vi "Cuboids example.vi"() -> ()   [LabVIEW 2013]
uses:
  Cuboids sub vis/Cuboid properties.ctl
  <vilib>/Utility/miscctls.llb/LV3DPointTypeDef.ctl
  <vilib>/Analysis/baseanly.llb/A x Vector.vi
  <vilib>/Analysis/_algsub.llb/Vector Norm.vi
  <vilib>/Analysis/_algsub.llb/Real Vector Norm.vi
  <vilib>/Analysis/baseanly.llb/Unit Vector.vi
  <vilib>/Analysis/baseanly.llb/Unit Vector (DBL).vi
  <vilib>/Analysis/baseanly.llb/Dot Product.vi
  <vilib>/Analysis/baseanly.llb/Real Dot Product.vi
  Cuboids sub vis/2D cross product.vi
  <vilib>/picture/3D Picture Control/Object/Add Object (no reference).vi
  <vilib>/picture/3D Picture Control/Object/Create Object (name).vi
  <vilib>/Analysis/Matrix/Numeric/Conversions/Array To Matrix - RA2.vi
  <vilib>/picture/3D Picture Control/NI_3D Picture Control.lvlib
  <vilib>/Analysis/NI_AALBase.lvlib
  <vilib>/Analysis/Matrix/NI_Matrix.lvlib
panel:
  in  "Reset view":bool
  in  "Stop Button":bool
  out "error out":errorcluster
  in  "Circle test min. dist.":dbl=100.0
  out "Minimum separation":dbl=0.19883626783883718
  out "Collision":bool
  in  "Rz2 (deg)":sgl(knob)=290.0 min=0 max=360 step=1 scale=0.0..360.0
  in  "Tx2, Ty2, Tz2":sgl[](array[slide])=[1.0, 0.0, 0.0] min=-5 max=5 step=0.1 scale=-5.0..5.0
  in  "Lx2, Ly2, Lz2":sgl[](array[slide])=[2.0, 0.2, 0.2] min=0 max=5 step=0.1 scale=0.0..5.0
  in  "Lx1, Ly1, Lz1":sgl[](array[slide])=[1.0, 1.0, 1.0] min=0 max=5 scale=0.0..5.0
  out "World":refnum<vi>(3d-picture)
  # "PN 30/08/2014"
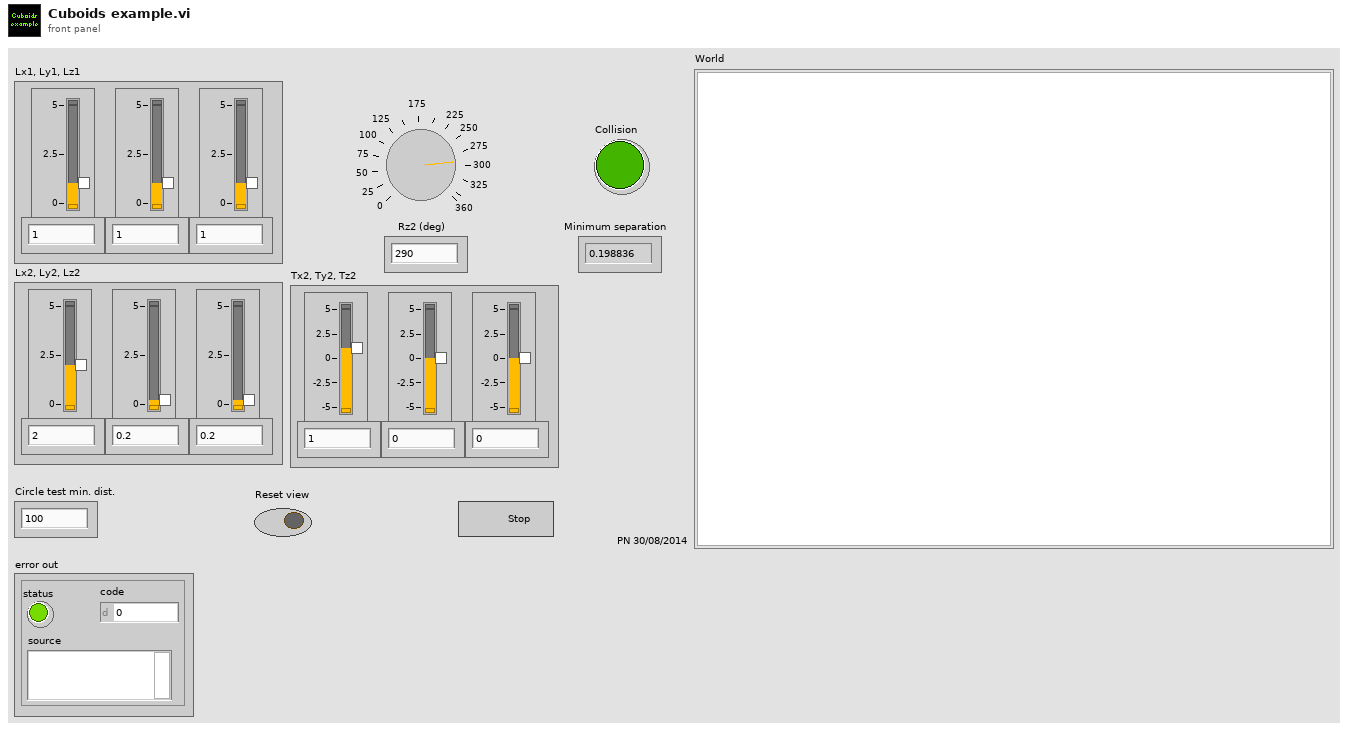
[diagram p1: front panel]
types:
  T1 = cluster{"Red":sgl, "Green":sgl, "Blue":sgl, "Alpha":sgl}
  T2 = typedef "LV3DPointTypeDef.ctl" = cluster{"X":sgl, "Y":sgl, "Z":sgl}
  T3 = typedef "Cuboid properties.ctl" = cluster{"Vertices (x, y)":dbl[][], "Zmin":dbl, "Zmax":dbl, "Centroid (x, y)":dbl[], "Radius":dbl, "Edge normals (x, y)":dbl[][], "Edge vectors (x, y)":dbl[][]}
  T4 = typedef "NI_Matrix.lvlib/RealMatrix.ctl" = dbl[][]
  T5 = cluster{"Vertical Pointer Slide":sgl, "Vertical Pointer Slide":sgl, "Vertical Pointer Slide":sgl}
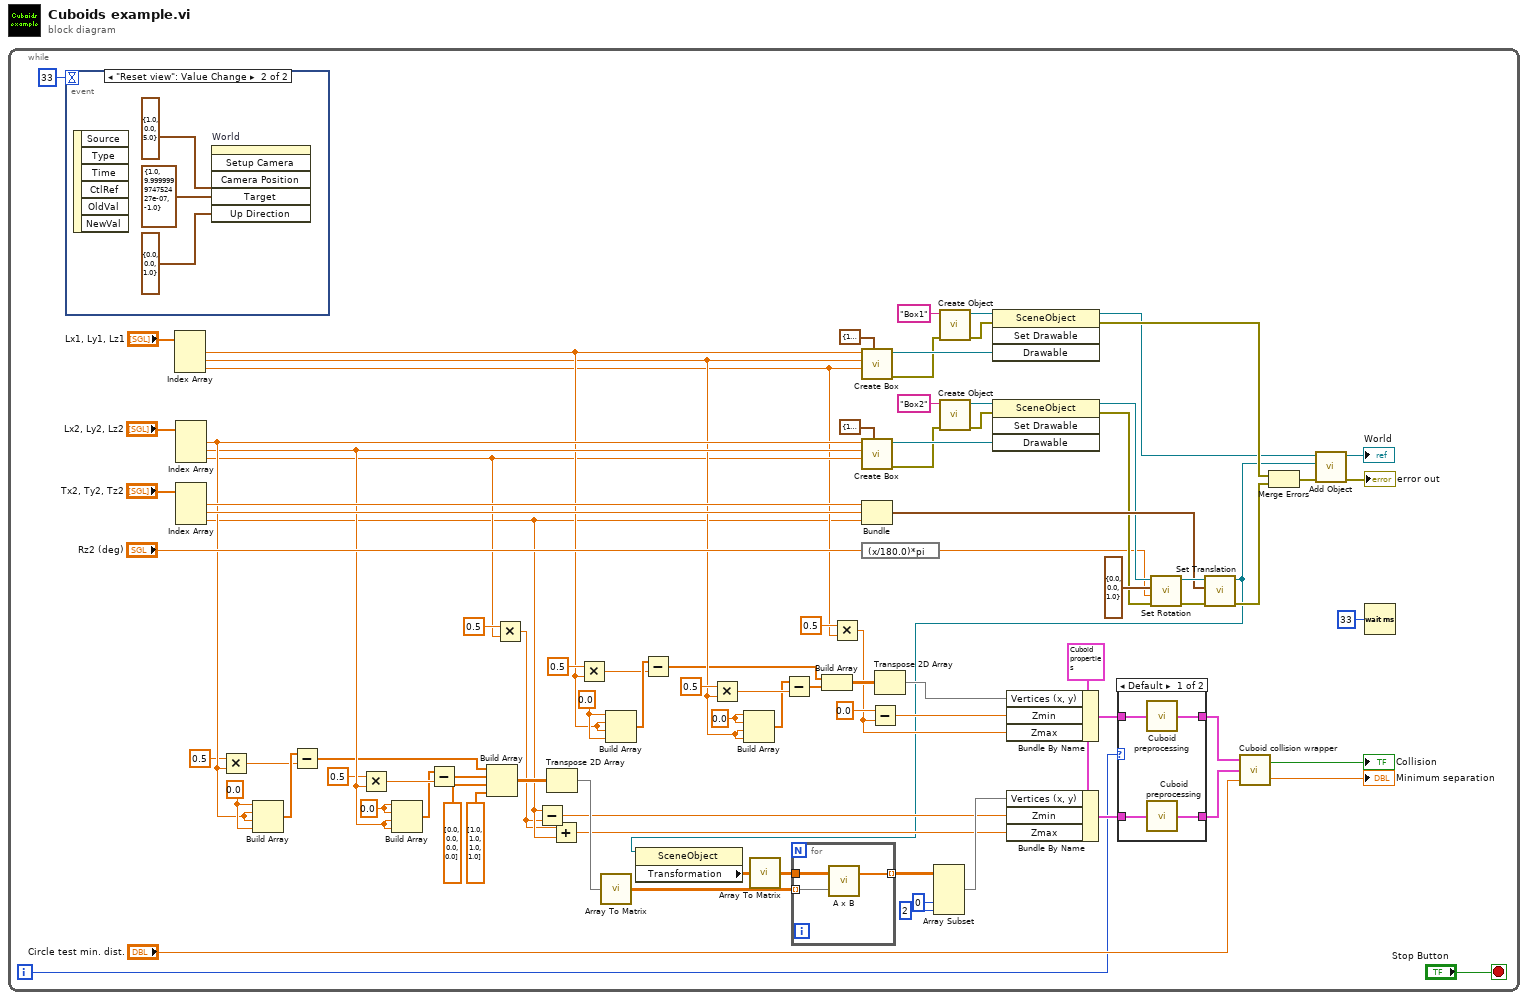
[diagram p0: block diagram]
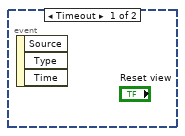
[diagram p2: hidden frame]
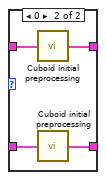
[diagram p3: hidden frame]
diagram:
  n1 = while {
    i -> [w16]
    stop <- "Stop Button" stop-if-true
    w53 = sgl 0.0 ("element")
    w54 = sgl 0.0 ("element")
    w55 = sgl 0.0 ("element")
    w56 = sgl 0.0 ("element")
    w67 = T3 {"Vertices (x, y)"=[[0.0, 0.0, 0.0], [1.0, 1.0, 0.0], [0.0, 1.0, 0.0], [1.0, 0.0, 0.0]], "Zmin"=0.0, "Zmax"=1.0, "Centroid (x, y)"=[0.0, 0.0, 0.0], "Radius"=0.0, "Edge normals (x, y)"=[[0.0, 0.0, 0.0], [0.0, 0.0, 0.0], [0.0, 0.0, 0.0], [0.0, 0.0, 0.0]], "Edge vectors (x, y)"=[[0.0, 0.0], [0.0, 0.0], [0.0, 0.0], [0.0, 0.0]]} ("Cuboid properties in")
    n2 = event shown="[1] \"Reset view\": Value Change" {
      selector: _ -> [_ _]
      dyn-events: _ -> [_ _]
      timeout: 33 -> [_ _]
      event Timeout {
        n3 = event-data() -> ()  [unwired: 1 in, 3 out]
      }
      event "Reset view": Value Change {
        n4 = event-data() -> ()  [unwired: 1 in, 6 out]
        n5 = invoke on="World" class="SceneGraphDisp (strict)" method="Setup Camera"("Camera Position"=T2 {"X"=1.0, "Y"=0.0, "Z"=5.0}, "Target"=T2 {"X"=1.0, "Y"=1e-06, "Z"=-1.0}, "Up Direction"=T2 {"X"=0.0, "Y"=0.0, "Z"=1.0}) -> ()  [unwired: 3 in, 6 out]
      }
    }
    n6 = Index Array(array="Lx1, Ly1, Lz1") -> (element #1=w33:sgl, element #2=w31:sgl, element #3=w9:sgl)  [unwired: 3 in]
    n7 = Index Array(array="Lx2, Ly2, Lz2") -> (element #1=w44:sgl, element #2=w42:sgl, element #3=w12:sgl)  [unwired: 3 in]
    n8 = Index Array(array="Tx2, Ty2, Tz2") -> (element #1=w64:sgl, element #2=w63:sgl, element #3=w5:sgl)  [unwired: 3 in]
    n9 = Multiply(x=sgl 0.5, y=w44) -> (x*y=w39:sgl)
    n10 = Build Array(w54, w44, w44, w54) -> (w40:sgl[])
    n11 = Subtract(x=w40, y=w39) -> (x-y=w38:sgl[])
    n12 = Multiply(x=sgl 0.5, y=w42) -> (x*y=w37:sgl)
    n13 = Build Array(w53, w53, w42, w42) -> (w36:sgl[])
    n14 = Subtract(x=w36, y=w37) -> (x-y=w35:sgl[])
    n15 = Build Array(w38, w35, sgl[] [0.0, 0.0, 0.0, 0.0], sgl[] [1.0, 1.0, 1.0, 1.0]) -> (w62:sgl[][])
    n16 = Multiply(x=sgl 0.5, y=w12) -> (x*y=w3:sgl)
    n17 = Subtract(x=w5, y=w3) -> (x-y=w4:sgl)
    n18 = Transpose 2D Array(2D array=w62) -> (transposed array=w24:sgl[][])
    n19 = Add(x=w3, y=w5) -> (x+y=w6:sgl)
    n20 = Multiply(x=sgl 0.5, y=w33) -> (x*y=w29:sgl)
    n21 = call-poly <vilib>:"Array To Matrix.vi"("Real 2D Array"=w24) -> ("Real Matrix"=w50:T4)
    n22 = Build Array(w56, w33, w33, w56) -> (w30:sgl[])
    n23 = Subtract(x=w30, y=w29) -> (x-y=w28:sgl[])
    n24 = Multiply(x=sgl 0.5, y=w31) -> (x*y=w27:sgl)
    n25 = Build Array(w55, w55, w31, w31) -> (w26:sgl[])
    n26 = Subtract(x=w26, y=w27) -> (x-y=w25:sgl[])
    n27 = Build Array(w28, w25) -> (w65:sgl[][])
    n28 = Multiply(x=sgl 0.5, y=w9) -> (x*y=w7:sgl)
    n29 = call <vilib>:"Create Box.vi"("Color"=T1 {"Red"=1.0, "Green"=1.0, "Blue"=1.0, "Alpha"=1.0}, "Length Z"=w9, "Length Y"=w31, "Length X"=w33) -> ("error out"=w82:errorcluster, "New Box Refnum"=w87:refnum<vi>)  [unwired: 6 in]
    n30 = call <vilib>:"Create Box.vi"("Color"=T1 {"Red"=1.0, "Green"=1.0, "Blue"=1.0, "Alpha"=1.0}, "Length Z"=w12, "Length Y"=w42, "Length X"=w44) -> ("error out"=w72:errorcluster, "New Box Refnum"=w83:refnum<vi>)  [unwired: 6 in]
    n31 = Bundle("Vertical Pointer Slide"=w64, "Vertical Pointer Slide"=w63, "Vertical Pointer Slide"=w5) -> (w79:T5)  [unwired: 1 in]
    n32 = expression code="(x/180.0)*pi" ("degrees to radians")("Rz2 (deg)") -> (w59:sgl)
    n33 = Subtract(x=sgl 0.0 ("element"), y=w7) -> (x-y=w8:sgl)
    n34 = Transpose 2D Array(2D array=w65) -> (transposed array=w61:sgl[][])
    n35 = call-poly <vilib>:"Create Object.vi"("error in (no error)"=w82, "Name"="Box1") -> ("error out"=w88:errorcluster, "Scene:New Object"=w89:refnum<vi>)  [unwired: 8 in]
    n36 = call-poly <vilib>:"Create Object.vi"("error in (no error)"=w72, "Name"="Box2") -> ("error out"=w71:errorcluster, "Scene:New Object"=w74:refnum<vi>)  [unwired: 8 in]
    n37 = invoke class="SceneObject" method="Set Drawable"(reference=w89, error in=w88, "Drawable"=w87) -> (reference out=w57:refnum<vi>, error out=w58:errorcluster)  [unwired: 1 in, 2 out]
    n38 = invoke class="SceneObject" method="Set Drawable"(reference=w74, error in=w71, "Drawable"=w83) -> (reference out=w75:refnum<vi>, error out=w76:errorcluster)  [unwired: 1 in, 2 out]
    n39 = Bundle By Name(cluster=w67, "Vertices (x, y)"=w61, "Zmin"=w8, "Zmax"=w7) -> (w68:T3)
    n40 = call <vilib>:"Set Rotation.vi"("error in (no error)"=w76, "Angle"=w59, "Axis"=cluster{"X":sgl, "Y":sgl, "Z":sgl} {"X"=0.0, "Y"=0.0, "Z"=1.0}, "Scene Object"=w75) -> ("error out"=w80:errorcluster, "Rotated Scene Object"=w81:refnum<vi>)  [unwired: 6 in]
    n41 = call <vilib>:"Set Translation.vi"("error in (no error)"=w80, "Translation"=w79, "Scene Object"=w81) -> ("error out"=w69:errorcluster, "Translated Object"=w1:refnum<vi>)  [unwired: 7 in]
    n42 = property class="SceneObject"(reference=w1) -> ("Transformation"=w52:sgl[][])  [unwired: 1 in, 2 out]
    n43 = call-poly <vilib>:"Array To Matrix.vi"("Real 2D Array"=w52) -> ("Real Matrix"=w17:T4)
    n44 = for {
      tunnel: w17 -> [w106]
      tunnel: w50 -> [w105] mode=indexing
      tunnel: [w104] -> w48 mode=indexing
      n45 = call-poly <vilib>:"A x B.vi"("Vector"=w105, "A"=w106) -> ("A x Vector"=w104:dbl[])  [unwired: 1 out]
    }
    n46 = Array Subset(array=w48, index (col)=0 ("index"), length (col)=2 ("length")) -> (w45:dbl[][])  [unwired: 2 in]
    n47 = Bundle By Name(cluster=w67, "Vertices (x, y)"=w45, "Zmin"=w4, "Zmax"=w6) -> (w66:T3)
    n48 = case shown="Default" w16 {
      tunnel: w68 -> [w99 w103]
      tunnel: w66 -> [w97 w102]
      tunnel: [w98 w101] -> w23
      tunnel: [w96 w100] -> w22
      frame Default {
        n49 = call "Cuboid preprocessing.vi"("Cuboid properties in"=w99) -> ("Cuboid properties out"=w98:T3)
        n50 = call "Cuboid preprocessing.vi"("Cuboid properties in"=w97) -> ("Cuboid properties out"=w96:T3)
      }
      frame 0 {
        n51 = call "Cuboid initial preprocessing.vi"("Cuboid properties in"=w103) -> ("Cuboid properties out"=w101:T3)
        n52 = call "Cuboid initial preprocessing.vi"("Cuboid properties in"=w102) -> ("Cuboid properties out"=w100:T3)
      }
    }
    n53 = call "Cuboid collision wrapper.vi"("Circle test min. dist."="Circle test min. dist.", "Cuboid 2"=w22, "Cuboid 1"=w23) -> ("Minimum separation"=→"Minimum separation":dbl, "Collision"=→"Collision":bool)
    n54 = Merge Errors(w58, w69) -> (w70:errorcluster)
    n55 = call-poly <vilib>:"Add Object.vi"("error in (no error)"=w70, "New Object In"=w1, "Scene Object In"=w57) -> ("error out"=→"error out":errorcluster, "Scene Object Out"=→"World":refnum<vi>)  [unwired: 7 in]
    n56 = Wait (ms)(milliseconds to wait=u32 33) -> ()  [unwired: 1 out]
  }
